vi "Get Location.vi"(11 "Class":refnum<class "Shield Wall.lvclass">) -> (0 "Post":T1, 2 "Ring":T2, 3 "Class":refnum<class "Shield Wall.lvclass">)   [LabVIEW 2015, in "Shield Wall.lvclass"]
uses:
  Shield Wall.lvclass
  Ring Enum.ctl
  Post Enum.ctl
  Shield Wall.lvclass/Shield Wall.ctl
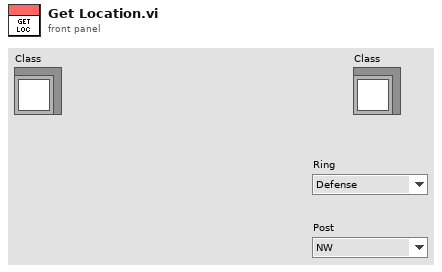
[diagram p1: front panel]
types:
  T1 = typedef "Shield Wall.lvclass/Post Enum.ctl" = enum16{"NW", "NNW", "NNE", "NE", "ENE", "ESE", "SE", "SSE", "SSW", "SW", "WSW", "WNW"}
  T2 = typedef "Shield Wall.lvclass/Ring Enum.ctl" = enum16{"Defense", "Fill", "Hold", "Spawn", "Replicate", "Inner"}
  T3 = typedef "Shield Wall.lvclass/DVR Cluster.ctl" = cluster{"N":i32, "E":i32, "S":i32, "W":i32, "Init":bool, "R":i32}
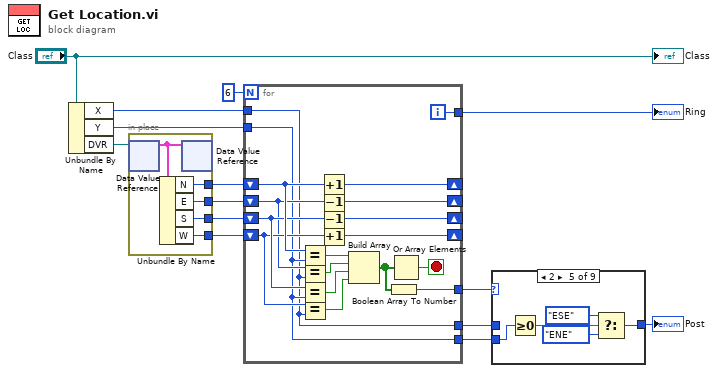
[diagram p0: block diagram]
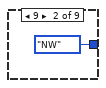
[diagram p3: hidden frame]
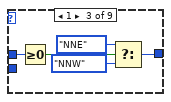
[diagram p4: hidden frame]
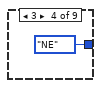
[diagram p5: hidden frame]
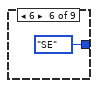
[diagram p6: hidden frame]
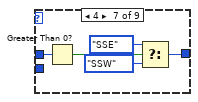
[diagram p7: hidden frame]
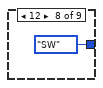
[diagram p8: hidden frame]
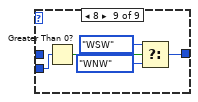
[diagram p9: hidden frame]
diagram:
  n1 = Unbundle By Name("Class") -> ("X"=w11:i32, "Y"=w12:i32, "DVR"=w13:refnum<data-value>)
  n2 = in-place {
    in-place-border: [w18] -> w10
    in-place-border: [w17] -> w9
    in-place-border: [w16] -> w8
    in-place-border: [w15] -> w7
    n3 = in-place-dvr #1(w13) -> (w19:T3)  [unwired: 1 out]
    n4 = Unbundle By Name(w19) -> ("N"=w18:i32, "E"=w17:i32, "S"=w16:i32, "W"=w15:i32)
    n5 = in-place-dvr #1(w19) -> ()  [unwired: 2 out]
  }
  n6 = for {
    N: 6 -> [_]
    tunnel: w12 -> [w21]
    tunnel: w11 -> [w20]
    tunnel: [w22] -> w6
    shift-right: [w32] -> _
    shift-left: w10 -> [w33]
    shift-right: [w26] -> _
    shift-left: w9 -> [w27]
    shift-right: [w30] -> _
    shift-left: w8 -> [w31]
    shift-right: [w28] -> _
    shift-left: w7 -> [w29]
    tunnel: [w23] -> w4
    tunnel: [w20] -> w3
    tunnel: [w21] -> w1
    i -> [w22]
    stop <- w25 stop-if-true
    n7 = Equal?(x=w33, y=w21) -> (x = y?=w37:bool)
    n8 = Equal?(x=w27, y=w20) -> (x = y?=w36:bool)
    n9 = Equal?(x=w31, y=w21) -> (x = y?=w35:bool)
    n10 = Equal?(x=w29, y=w20) -> (x = y?=w34:bool)
    n11 = Increment(x=w33) -> (x+1=w32:i32)
    n12 = Decrement(x=w27) -> (x-1=w26:i32)
    n13 = Decrement(x=w31) -> (x-1=w30:i32)
    n14 = Increment(x=w29) -> (x+1=w28:i32)
    n15 = Build Array(w37, w36, w35, w34) -> (w24:bool[])
    n16 = Boolean Array To Number(Boolean array=w24) -> (number=w23:u32)
    n17 = Or Array Elements(Boolean array=w24) -> (logical OR=w25:bool)
  }
  "Ring" <- w6
  n18 = case shown="2" w4 {
    tunnel: w3 -> [_ _ w43 _ _ _ w55 _ _]
    tunnel: [_ Post_Enum."NW" ("Post") w39 Post_Enum."NE" ("Post") w46 Post_Enum."SE" ("Post") w51 Post_Enum."SW" ("Post") w58] -> w2
    tunnel: w1 -> [_ _ _ _ w45 _ _ _ w57]
    frame Default {
    }
    frame 9 {
    }
    frame 1 {
      n19 = Greater Or Equal To 0?(x=w43) -> (x >= 0?=w42:bool)
      n20 = Select(t=Post_Enum."NNE" ("Post"), s=w42, f=Post_Enum."NNW" ("Post")) -> (s? t:f=w39:T1)
    }
    frame 3 {
    }
    frame 2 {
      n21 = Greater Or Equal To 0?(x=w45) -> (x >= 0?=w49:bool)
      n22 = Select(t=Post_Enum."ESE" ("Post"), s=w49, f=Post_Enum."ENE" ("Post")) -> (s? t:f=w46:T1)
    }
    frame 6 {
    }
    frame 4 {
      n23 = Greater Than 0?(x=w55) -> (x > 0?=w54:bool)
      n24 = Select(t=Post_Enum."SSE" ("Post"), s=w54, f=Post_Enum."SSW" ("Post")) -> (s? t:f=w51:T1)
    }
    frame 12 {
    }
    frame 8 {
      n25 = Greater Than 0?(x=w57) -> (x > 0?=w61:bool)
      n26 = Select(t=Post_Enum."WSW" ("Post"), s=w61, f=Post_Enum."WNW" ("Post")) -> (s? t:f=w58:T1)
    }
  }
  "Post" <- w2
  "Class" <- "Class"
